vi "CfgManager Test Launcher.vi"() -> ()   [LabVIEW 2013]
uses:
  Cache/ConfigManager.Cache.lvclass
  Manager/ConfigManager.lvclass
panel:
  out "keys listed":string[](array[string])
  out "keys written":string[](array[string])
  out "Values":variant[](array[variant])
  out "keys read":string[](array[string])
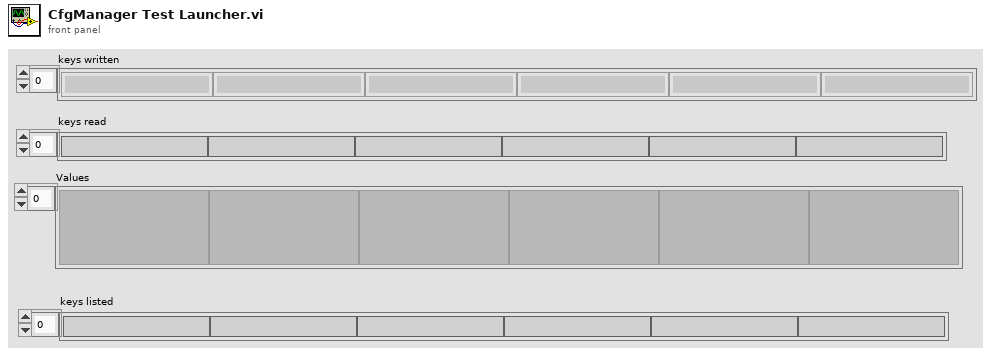
[diagram p1: front panel]
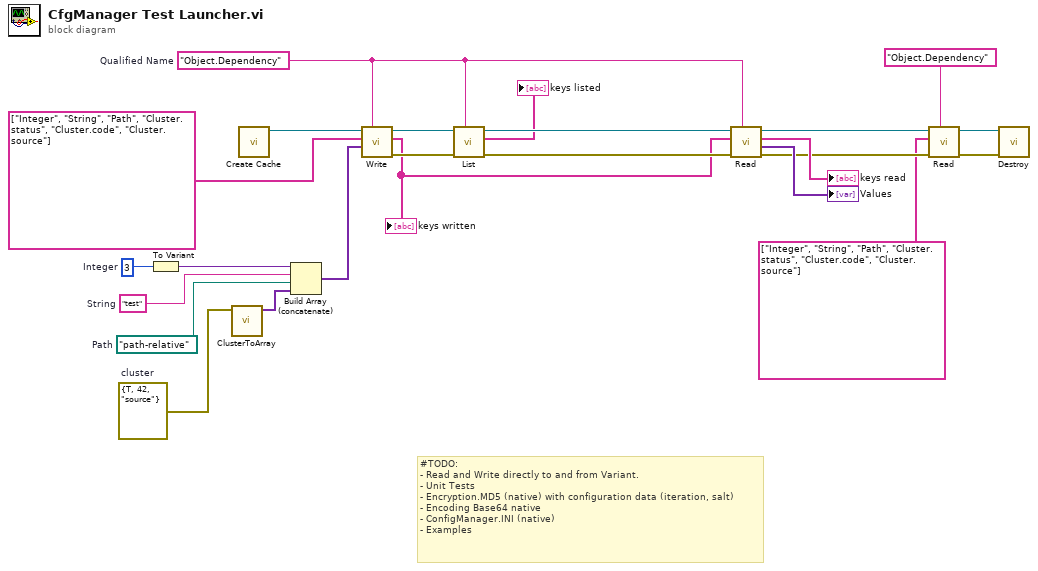
[diagram p0: block diagram]
diagram:
  w12 = "Object.Dependency"  # Qualified Name
  w10 = errorcluster {"status"=TRUE, "code"=42, "source"="source"}  # cluster
  w18 = path "path-relative"  # Path
  w19 = "test"  # String
  w21 = 3  # Integer
  # "#TODO: \n- Read and Write directly to and from Variant.\n- Unit Tests\n- Encryption.MD5 (native) with configuration data (iteration, salt)\n- Encoding Base64 native\n- ConfigManager.INI (native)\n- Examples"
  n1 = To Variant(anything=w21) -> (Variant=w20:variant)
  n2 = call "ClusterToArray.vi"("Cluster"=w10) -> ("Array"=w9:variant[])  [unwired: 10 in]
  n3 = call "Create Cache.vi"() -> ("ConfigManager.Cache"=w22:refnum<class "ConfigManager.Cache.lvclass">)  [unwired: 11 in]
  n4 = Build Array (concatenate)(w20, w19, w18, w9) -> (w17:variant[])
  n5 = call "Write.vi"("Qualified Name"=w12, "Values"=w17, "keys"=string[] ["Integer", "String", "Path", "Cluster.status", "Cluster.code", "Cluster.source"] ("keys written"), "ConfigManager in"=w22) -> ("error out"=w14:errorcluster, "keys dup"=w7:string[], "ConfigManager out"=w16:refnum<class "ConfigManager.Cache.lvclass">)  [unwired: 5 in]
  "keys written" <- w7
  n6 = call "List.vi"("Qualified Name"=w12, "error in (no error)"=w14, "ConfigManager in"=w16) -> ("error out"=w13:errorcluster, "Keys"=→"keys listed":string[], "ConfigManager out"=w15:refnum<class "ConfigManager.Cache.lvclass">)  [unwired: 6 in]
  n7 = call "Read.vi"("Qualified Name"=w12, "error in (no error)"=w13, "keys in"=w7, "ConfigManager in"=w15) -> ("error out"=w4:errorcluster, "Values"=→"Values":variant[], "keys"=→"keys read":string[], "ConfigManager out"=w6:refnum<class "ConfigManager.Cache.lvclass">)  [unwired: 4 in]
  n8 = call "Read.vi"("Qualified Name"="Object.Dependency" ("Name"), "error in (no error)"=w4, "keys in"=string[] ["Integer", "String", "Path", "Cluster.status", "Cluster.code", "Cluster.source"] ("keys written"), "ConfigManager in"=w6) -> ("error out"=w3:errorcluster, "ConfigManager out"=w5:refnum<class "ConfigManager.Cache.lvclass">)  [unwired: 4 in, 2 out]
  n9 = call-dynamic "Destroy.vi"("error in (no error)"=w3, "ConfigManager.Cache in"=w5) -> ()  [unwired: 8 in, 2 out]
